vi "filereader.vi"() -> ()   [LabVIEW 2015]
panel:
  in  "Path":path
  out "String Read":string
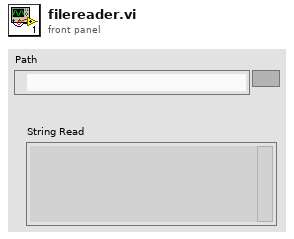
[diagram p1: front panel]
types:
  T1 = enum16{"open", "open or create", "create or replace", "create", "open (read only)"}
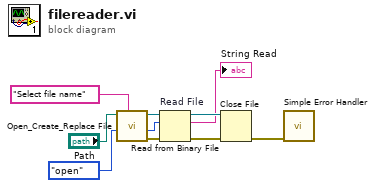
[diagram p0: block diagram]
diagram:
  n1 = call <vilib>:"Open_Create_Replace File.vi"("prompt"="Select file name", "function (open:0)"=T1."open", "file path"="Path") -> ("error out"=w7:errorcluster, "file size (bytes)"=w3:i32, "refnum"=w6:refnum<file>)  [unwired: 5 in, 1 out]
  n2 = Read from Binary File "Read File"(8:w7, 10:w3, 11:w6) -> (0:w4:errorcluster, 2:→"String Read":string, 3:w5:refnum<file>)  [unwired: 3 in, 1 out]
  n3 = Close File(refnum=w5, error in=w4) -> (error out=w10:errorcluster)  [unwired: 1 out]
  n4 = call <vilib>:"Simple Error Handler.vi"("error in (no error)"=w10) -> ()  [unwired: 4 in, 5 out]
